vi "Construct Test Result.vi"(8 "error in (no error)":errorcluster, 11 "Test Case":refnum<class "Test Case.lvclass">) -> (0 "error out":errorcluster, 3 "Test Result":refnum<class "Test Result.lvclass">)   [LabVIEW 2017, in "Test Result.lvclass"]
uses:
  Test Result.lvclass
  Test Case/Test Case.lvclass
  Test Result.lvclass/Test Result.ctl
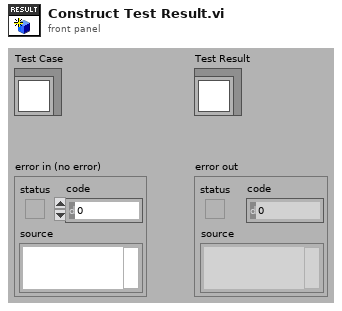
[diagram p1: front panel]
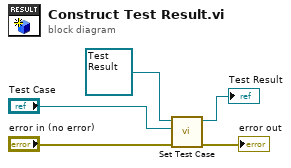
[diagram p0: block diagram]
diagram:
  n1 = call "Set Test Case.vi"("error in (no error)"="error in (no error)", "Test Case"="Test Case", "Test Result in"=refnum<class "Test Result.lvclass"> refnum) -> ("error out"=→"error out":errorcluster, "Test Result out"=→"Test Result":refnum<class "Test Result.lvclass">)  [unwired: 7 in]
